vi "Controller Response Matrix Measurement Loop.vi"(7 "Sync Objects":T1, 8 "error in (no error)":errorcluster, 11 "FOFB Configuration":T4={"FOFB Parameters"={"Network"={"FOFB Controller IP"="", "LNLS Control Network IP"="", "LNLS Control Network Power Supplies TCP Port"=0, "LNLS Control Network FOFB Configuration TCP Port"=0, "LNLS Control Network BPMs TCP Port"=0, "Data Server TCP Port"=0, "Monitoring Data TCP Port"=0, "Configuration GUI TCP Port"=0, "Storage Data TCP Port"=0, "TCP Listening Timeout"=0, "Request Setpoints Rate"=0}, "Fast Acquisition"={"Acquisition Period"=0, "Data Buffer Size"=0, "Monitoring Period"=0}, "Response Matrix Measurement"={"Step Amplitude"=0.0, "Time Between Steps"=0, "Step Duration"=0, "Number of Averages"=0}, "Correction Algorithm"={"Correction Period"=0, "Reference Orbit Path"=path "", "Response Matrix Path"=path "", "Correction Matrix Path"=path "", "PID Horizontal Gain"=0.0, "PID Vertical Gain"=0.0, "PID Horizontal Integral Time"=0.0, "PID Vertical Integral Time"=0.0, "PID Horizontal Derivative Time"=0.0, "PID Vertical Derivative Time"=0.0, "Beam Current FOFB Threshold"=0.0, "Decouple H-V"=FALSE, "Use Additional BPM LPF"=FALSE, "BPM LPF Cutoff"=0.0}, "Acquisition Network"=[], "Actuation Network"=[]}, "Number of Acquisition Chassis"=0, "Number of Actuation Chassis"=0, "Number of BPM Readings"=0, "BPM Reading Names"=[], "Selected BPM Readings"=[0, 1, 2, 3, 4, 5, 6, 7, 8, 9, 10, 11, 12, 13, 14, 15, 16, 17, 18, 19, 20, 21, 22, 23, 24, 25, 26, 27, 28, 29, 30, 31, 32, 33, 34, 35, 36, 37, 38, 39, 40, 41, 42, 43, 44, 45, 46, 47, 48, 49], "Number of Correctors"=0, "Corrector Names"=[], "Selected Correctors"=[0, 1, 2, 3, 4, 5, 6, 7, 8, 9, 10, 11, 12, 13, 14, 15, 16, 17, 18, 19, 20, 21, 22, 23, 24, 25, 26, 27, 28, 29, 30, 31, 32, 33, 34, 35, 36, 37, 38, 39, 40, 41, 42, 43, 44, 45, 46, 47, 48, 49], "Reference Orbit"=[], "Response Matrix"=[], "Correction Matrix"=[], "Acquisition Chassis Names"=[], "Actuation Chassis Names"=[], "Acquisition Variables"=[], "Actuation Variables"=[], "PS Matrix Mapping"=[], "Inverse PS Matrix Mapping"=[], "BPM Matrix Mapping"=[], "Inverse BPM Matrix Mapping"=[], "Response Matrix Beam Energy (MeV)"=0.0, "PID Parameters"=[], "BPM Planes"=[], "Corrector Planes"=[], "RMM Step Factor"=[]}) -> (0 "error out":errorcluster)   [LabVIEW 2011, in "Controller VIs.lvlib"]
uses:
  Controller VIs.lvlib
  Types Definitions/Type FOFB Configuration.ctl
  Types Definitions/Type FOFB Parameters.ctl
  Types Definitions/Type Network Configuration.ctl
  Types Definitions/Type FA Configuration.ctl
  Types Definitions/Type Response Matrix Measurement Configuration.ctl
  Types Definitions/Type Correction Algorithm Configuration.ctl
  Types Definitions/Type Acquisition Network Configuration.ctl
  Types Definitions/Type Actuation Network Configuration.ctl
  Types Definitions/Type PID Parameters.ctl
  Types Definitions/Type Synchronization Objects.ctl
  Types Definitions/Type Blocking Synchronization Objects.ctl
  Types Definitions/Type Monitoring Data.ctl
  Types Definitions/Type Operation Mode State.ctl
  Types Definitions/Type Diagnostics Data.ctl
  Types Definitions/Type CPU Loads Array.ctl
  Types Definitions/Type CPU Loads.ctl
  Types Definitions/Type Non-blocking Synchronization Objects.ctl
  Types Definitions/Type FOFB Variables.ctl
  Types Definitions/Type Actuation State.ctl
  <vilib>/Platform/TimedLoop/XDataNode/timing_clust.ctl
  <vilib>/Platform/TimedLoop/XDataNode/nitl_modes.ctl
  <vilib>/Platform/TimedLoop/XDataNode/wakeup.ctl
  Controller Global Variables/Monitoring Data.vi
  <vilib>/Platform/TimedLoop/XDataNode/XDataNode.xnode
  File VIs.lvlib
  Controller Global Variables.lvlib
  Controller Global Variables/LNLS Control FOFB Configuration Out.vi
  <vilib>/Platform/TimedLoop/XDataNode/XDNodeRunTimeDep.lvlib
  Type Definitions.lvlib
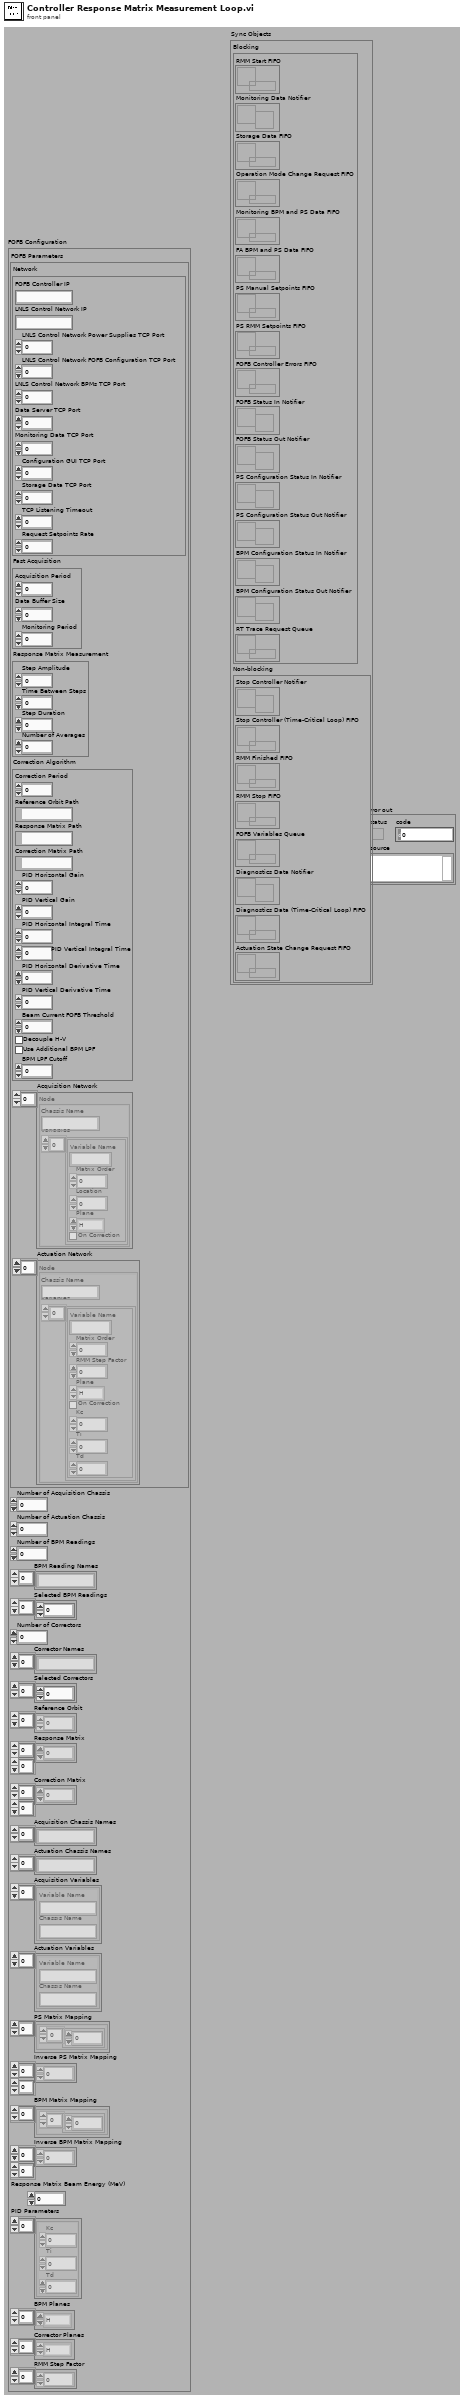
[diagram p1: front panel]
types:
  T1 = typedef "Type Definitions.lvlib/Type Synchronization Objects.ctl" = cluster{"Blocking":T2, "Non-blocking":T3}
  T2 = typedef "Type Definitions.lvlib/Type Blocking Synchronization Objects.ctl" = cluster{"RMM Start FIFO":refnum<k33>, "Monitoring Data Notifier":refnum<notifier>, "Storage Data FIFO":refnum<queue>, "Operation Mode Change Request FIFO":refnum<k33>, "Monitoring BPM and PS Data FIFO":refnum<k33>, "FA BPM and PS Data FIFO":refnum<k33>, "PS Manual Setpoints FIFO":refnum<k33>, "PS RMM Setpoints FIFO":refnum<k33>, "FOFB Controller Errors FIFO ":refnum<k33>, "FOFB Status In Notifier":refnum<notifier>, "FOFB Status Out Notifier":refnum<notifier>, "PS Configuration Status In Notifier":refnum<notifier>, "PS Configuration Status Out Notifier":refnum<notifier>, "BPM Configuration Status In Notifier":refnum<notifier>, "BPM Configuration Status Out Notifier":refnum<notifier>, "RT Trace Request Queue":refnum<queue>}
  T3 = typedef "Type Definitions.lvlib/Type Non-blocking Synchronization Objects.ctl" = cluster{"Stop Controller Notifier":refnum<notifier>, "Stop Controller (Time-Critical Loop) FIFO":refnum<k33>, "RMM Finished FIFO":refnum<k33>, "RMM Stop FIFO":refnum<k33>, "FOFB Variables Queue":refnum<queue>, "Diagnostics Data Notifier":refnum<notifier>, "Diagnostics Data (Time-Critical Loop) FIFO":refnum<k33>, "Actuation State Change Request FIFO":refnum<k33>}
  T4 = typedef "Type Definitions.lvlib/Type FOFB Configuration.ctl" = cluster{"FOFB Parameters":T5, "Number of Acquisition Chassis":i32, "Number of Actuation Chassis":i32, "Number of BPM Readings":i32, "BPM Reading Names":string[], "Selected BPM Readings":u32[], "Number of Correctors":i32, "Corrector Names":string[], "Selected Correctors":u32[], "Reference Orbit":dbl[], "Response Matrix":dbl[][], "Correction Matrix":dbl[][], "Acquisition Chassis Names":string[], "Actuation Chassis Names":string[], "Acquisition Variables":cluster{"Variable Name":string, "Chassis Name":string}[], "Actuation Variables":cluster{"Variable Name":string, "Chassis Name":string}[], "PS Matrix Mapping":cluster{u32[]}[], "Inverse PS Matrix Mapping":u32[][], "BPM Matrix Mapping":cluster{u32[]}[], "Inverse BPM Matrix Mapping":u32[][], "Response Matrix Beam Energy (MeV)":dbl, "PID Parameters":T12[], "BPM Planes":enum8{"H", "V"}[], "Corrector Planes":enum8{"H", "V"}[], "RMM Step Factor":dbl[]}
  T5 = typedef "Type Definitions.lvlib/Type FOFB Parameters.ctl" = cluster{"Network":T6, "Fast Acquisition":T7, "Response Matrix Measurement":T8, "Correction Algorithm":T9, "Acquisition Network":T10, "Actuation Network":T11}
  T6 = typedef "Type Definitions.lvlib/Type Network Configuration.ctl" = cluster{"FOFB Controller IP":string, "LNLS Control Network IP":string, "LNLS Control Network Power Supplies TCP Port":u16, "LNLS Control Network FOFB Configuration TCP Port":u16, "LNLS Control Network BPMs TCP Port":u16, "Data Server TCP Port":u16, "Monitoring Data TCP Port":u16, "Configuration GUI TCP Port":u16, "Storage Data TCP Port":u16, "TCP Listening Timeout":i32, "Request Setpoints Rate":u16}
  T7 = typedef "Type Definitions.lvlib/Type FA Configuration.ctl" = cluster{"Acquisition Period":u32, "Data Buffer Size":u32, "Monitoring Period":u32}
  T8 = typedef "Type Definitions.lvlib/Type Response Matrix Measurement Configuration.ctl" = cluster{"Step Amplitude":dbl, "Time Between Steps":u32, "Step Duration":u32, "Number of Averages":u32}
  T9 = typedef "Type Definitions.lvlib/Type Correction Algorithm Configuration.ctl" = cluster{"Correction Period":u32, "Reference Orbit Path":path, "Response Matrix Path":path, "Correction Matrix Path":path, "PID Horizontal Gain":dbl, "PID Vertical Gain":dbl, "PID Horizontal Integral Time":dbl, "PID Vertical Integral Time":dbl, "PID Horizontal Derivative Time":dbl, "PID Vertical Derivative Time":dbl, "Beam Current FOFB Threshold":dbl, "Decouple H-V":bool, "Use Additional BPM LPF":bool, "BPM LPF Cutoff":dbl}
  T10 = typedef "Type Definitions.lvlib/Type Acquisition Network Configuration.ctl" = cluster{"Chassis Name":string, "Variables":cluster{"Variable Name":string, "Matrix Order":u32, "Location":dbl, "Plane":enum8{"H", "V"}, "On Correction":bool}[]}[]
  T11 = typedef "Type Definitions.lvlib/Type Actuation Network Configuration.ctl" = cluster{"Chassis Name":string, "Variables":cluster{"Variable Name":string, "Matrix Order":u32, "RMM Step Factor":dbl, "Plane":enum8{"H", "V"}, "On Correction":bool, "Kc":dbl, "Ti":dbl, "Td":dbl}[]}[]
  T12 = typedef "Type Definitions.lvlib/Type PID Parameters.ctl" = cluster{"Kc":fxp<+/-,16,8>, "Ti":fxp<+/-,16,8>, "Td":fxp<+/-,16,8>}
  T13 = typedef "XDNodeRunTimeDep.lvlib/timing_clust.ctl" = cluster{"Expected End [f-1]":u64, "Actual End [f-1]":u64, "Finished Late? [f-1]":bool, "Expected End [i-1]":u64, "Actual End [i-1]":u64, "Finished Late? [i-1]":bool, "Expected Start [i]":u64, "Actual Start [i]":u64, "Expected Start [f]":u64, "Actual Start [f]":u64, "Source Name":string, "Structure Name":string, "Period":i64, "Deadline":i64, "Offset":i64, "Start":i64, "Priority":i32, "Timeout":i32, "Mode":T14, "Wakeup Reason":T15, "Error":errorcluster, "Source Type":string, "Secondary Source Type":string, "Global End Time":u64, "Global Start Time":u64, "Frame Duration":u64, "Iteration Duration":u64, "Assigned CPU":i32, "I/O Scan Engine Mode":u32}
  T14 = typedef "XDNodeRunTimeDep.lvlib/nitl_modes.ctl" = enum32{"No Change", "Process missed periods, maintain original phase", "Discard missed periods, maintain original phase", "Process missed periods, ignore original phase", "Discard missed periods, ignore original phase"}
  T15 = typedef "XDNodeRunTimeDep.lvlib/wakeup.ctl" = enum32{"Normal", "Aborted", "Asynchronous wakeup", "Timing source error", "Timed loop error", "Timeout"}
  T16 = typedef "Type Definitions.lvlib/Type Monitoring Data.ctl" = cluster{"Timestamp":timestamp, "BPM Readings":dbl[], "PS Readings":dbl[], "PS FOFB Setpoints":dbl[], "PS Status per Rack":u8[], "PS ON-OFF per Rack":u8[], "Operation Mode":T17, "Diagnostics Data":T18, "Controller Status Table":i32[]}
  T17 = typedef "Type Definitions.lvlib/Type Operation Mode State.ctl" = enum8{"Idle Mode", "Manual Mode", "FOFB Mode", "RMM Mode"}
  T18 = typedef "Type Definitions.lvlib/Type Diagnostics Data.ctl" = cluster{"Time-Critical Loop Missed Iterations":u32, "Time-Critical Loop Execution Time (usec)":u32, "Available Memory (bytes)":u32, "CPU Loads Array":T19}
  T19 = typedef "Type Definitions.lvlib/Type CPU Loads Array.ctl" = T20[]
  T20 = typedef "Type Definitions.lvlib/Type CPU Loads.ctl" = cluster{"Total (%)":dbl, "Time Critical (%)":dbl, "Timed Structures (%)":dbl, "High (%)":dbl, "Above Normal (%)":dbl, "Normal (%)":dbl, "Background (%)":dbl, "Idle (%)":dbl, "ISR (%)":dbl}
  T21 = typedef "Type Definitions.lvlib/Type Control FOFB Configuration Out.ctl" = cluster{"Status":u16, "Operation Mode":T17, "PID Horizontal Gain":sgl, "PID Vertical Gain":sgl, "PID Horizontal Integral Time":sgl, "PID Vertical Integral Time":sgl, "PID Horizontal Derivative Time":sgl, "PID Vertical Derivative Time":sgl, "RMS Horizontal Distortion":dbl, "RMS Vertical Distortion":dbl, "Timestamp":u64}
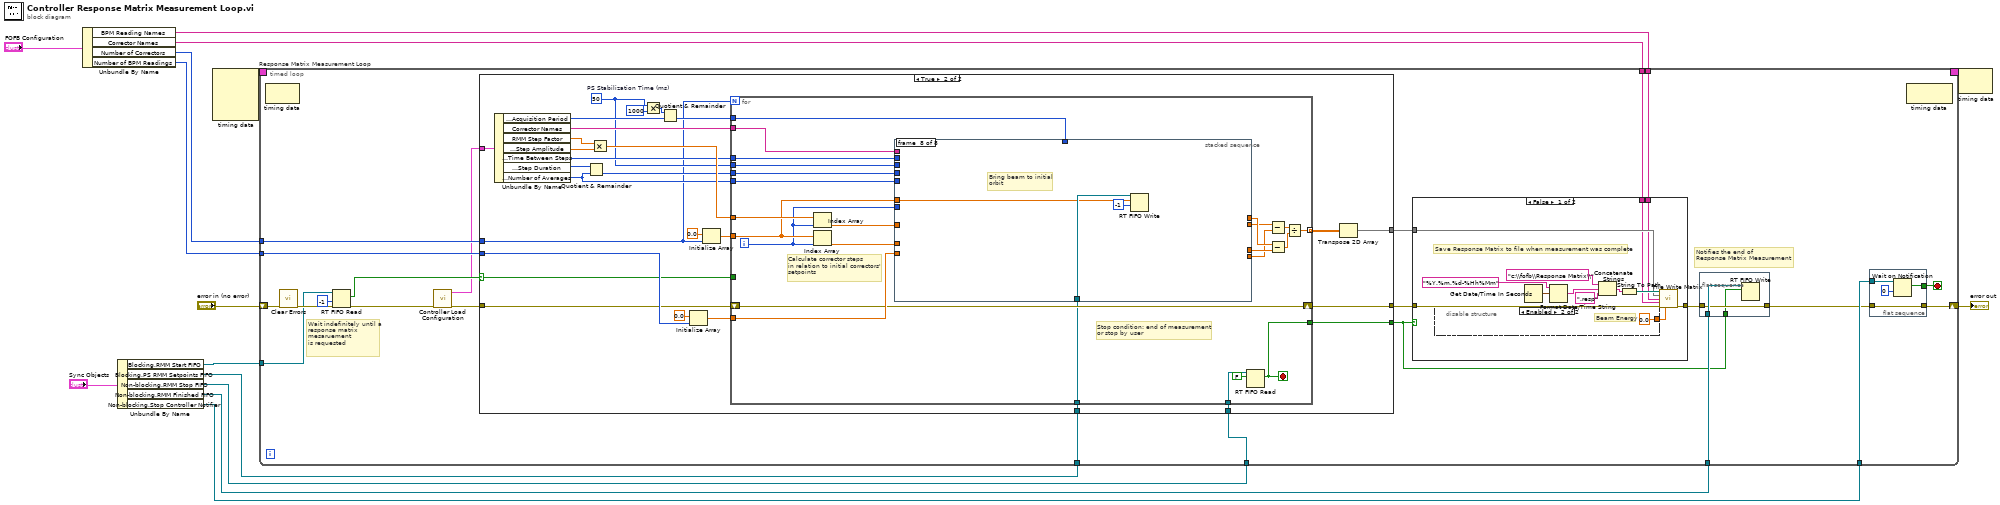
[diagram p0: block diagram]
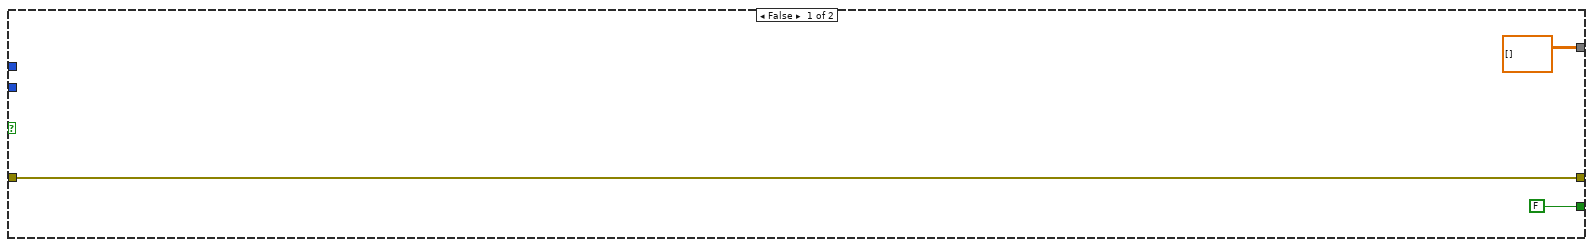
[diagram p2: hidden frame]
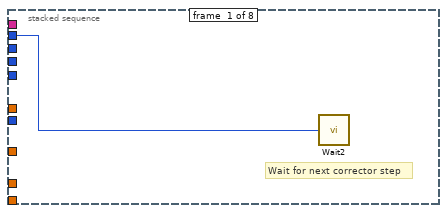
[diagram p3: hidden frame]
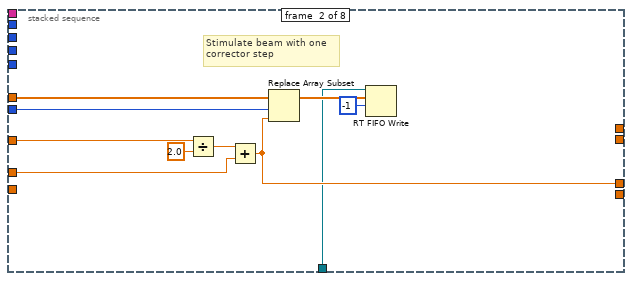
[diagram p4: hidden frame]
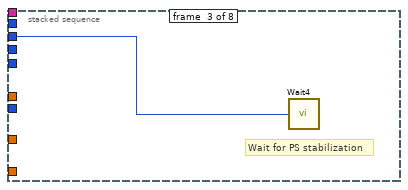
[diagram p5: hidden frame]
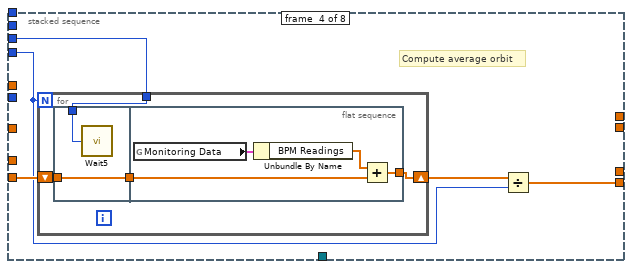
[diagram p6: hidden frame]
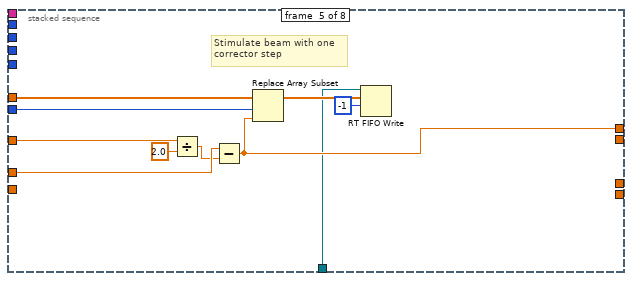
[diagram p7: hidden frame]
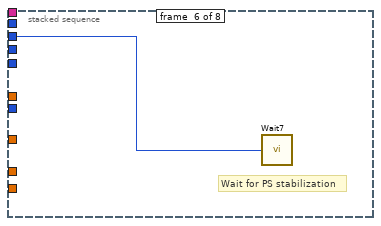
[diagram p8: hidden frame]
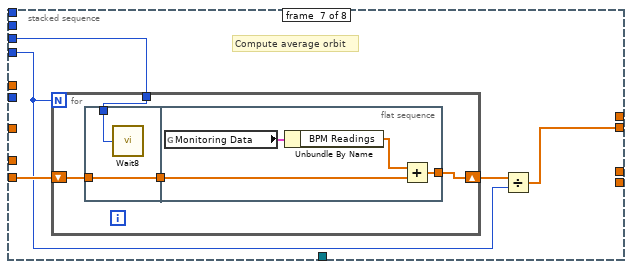
[diagram p9: hidden frame]
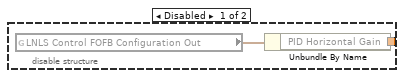
[diagram p10: hidden frame]
diagram:
  n1 = Unbundle By Name("FOFB Configuration") -> ("BPM Reading Names"=w7:string[], "Corrector Names"=w6:string[], "Number of Correctors"=w9:i32, "Number of BPM Readings"=w8:i32)
  n2 = Unbundle By Name("Sync Objects") -> ("Blocking.RMM Start FIFO"=w5:refnum<k33>, "Blocking.PS RMM Setpoints FIFO"=w3:refnum<k33>, "Non-blocking.RMM Stop FIFO"=w10:refnum<k33>, "Non-blocking.RMM Finished FIFO"=w12:refnum<k33>, "Non-blocking.Stop Controller Notifier"=w11:refnum<notifier>)
  n3 = node-c288() -> (w2:T13)  [unwired: 4 in]
  n4 = timed-loop "Response Matrix Measurement Loop" {
    shift-right: [w26] -> w15
    shift-left: "error in (no error)" -> [w21]
    tunnel: w9 -> [w38]
    tunnel: w8 -> [w23]
    tunnel: w7 -> [w37]
    tunnel: w6 -> [w36]
    tunnel: w12 -> [w31]
    tunnel: w11 -> [w35]
    tunnel: w10 -> [w32]
    tunnel: w5 -> [w18]
    tunnel: w3 -> [w24]
    timing: w2 -> [_]
    timing-out: [_] -> w1
    stop <- w27 stop-if-true
    # "Notifies the end of\nResponse Matrix Measurement"
    # "Wait indefinitely until a response matrix mesaruement\nis requested"
    n5 = node-c288() -> ()  [unwired: 1 in, 1 out]
    n6 = call <vilib>:"Clear Errors.vi"("error in (no error)"=w21) -> ("error out"=w19:errorcluster)  [unwired: 6 in]
    n7 = RT FIFO Read(0:w18, 2:-1 ("timeout in ms (-1)"), 3:w19) -> (9:w28:bool, 11:w16:errorcluster)  [unwired: 1 in, 3 out]
    n8 = call "Controller Load Configuration.vi"("error in (no error)"=w16) -> ("error out"=w17:errorcluster, "FOFB Configuration"=w22:T4)  [unwired: 9 in]
    n9 = case shown="True" w28 {
      selector: w28 -> [_ w52]
      tunnel: w17 -> [w50 w66]
      tunnel: [w50 w72] -> w34
      tunnel: [FALSE ("Calculation Stopped?") w71] -> w29
      tunnel: [dbl[][] [] ("Response Matrix") w69] -> w33
      tunnel: w38 -> [_ w51]
      tunnel: w23 -> [_ w68]
      tunnel: w32 -> [_ w63]
      tunnel: w22 -> [_ w62]
      tunnel: w24 -> [_ w59]
      frame False {
      }
      frame True {
        w53 = u32 50  # PS Stabilization Time (ms)
        n10 = Unbundle By Name(w62) -> ("FOFB Parameters.Fast Acquisition.Acquisition Period"=w58:u32, "Corrector Names"=w60:string[], "RMM Step Factor"=w61:dbl[], "FOFB Parameters.Response Matrix Measurement.Step Amplitude"=w77:dbl, "FOFB Parameters.Response Matrix Measurement.Time Between Steps"=w56:u32, "FOFB Parameters.Response Matrix Measurement.Step Duration"=w65:u32, "FOFB Parameters.Response Matrix Measurement.Number of Averages"=w64:u32)
        n11 = Quotient & Remainder(x=w65, y=w64) -> (floor(x/y)=w73:u32)  [unwired: 1 out]
        n12 = Multiply(x=w61, y=w77) -> (x*y=w76:dbl[])
        n13 = Multiply(x=w53, y=u32 1000) -> (x*y=w57:u32)
        n14 = Quotient & Remainder(x=w57, y=w58) -> (floor(x/y)=w54:u32)  [unwired: 1 out]
        n15 = Initialize Array(0.0 ("element"), w68) -> (w74:dbl[])
        n16 = Initialize Array(0.0 ("element"), w51) -> (w67:dbl[])
        n17 = for {
          N: w51 -> [_]
          tunnel: w67 -> [w101]
          tunnel: w76 -> [w102]
          shift-right: [w87] -> w72
          shift-left: w66 -> [w87]
          tunnel: w64 -> [w100]
          tunnel: w74 -> [w99]
          tunnel: w73 -> [w98]
          tunnel: [w86] -> w70 mode=indexing
          tunnel: w56 -> [w89]
          tunnel: [w79] -> w71
          tunnel: w53 -> [w88]
          tunnel: w63 -> [w85]
          tunnel: w60 -> [w84]
          tunnel: w59 -> [w82]
          tunnel: w54 -> [w81]
          tunnel: w52 -> [_]
          i -> [w80]
          stop <- w79 stop-if-true
          # "Stop condition: end of measurement\nor stop by user"
          # "Calculate corrector steps\nin relation to initial correctors'\nsetpoints"
          n18 = Index Array(array=w102, index=w80) -> (element=w91:dbl)
          n19 = Index Array(array=w101, index=w80) -> (element=w90:dbl)
          n20 = stacked-sequence {
            tunnel: w101 -> [_ w109 _ _ w139 _ _ w156]
            tunnel: [_ _ _ _ w133 _ _ _] -> w94
            tunnel: [_ _ _ _ _ _ w141 _] -> w92
            tunnel: w100 -> [_ _ _ w115 _ _ w142 _]
            tunnel: [_ _ _ w118 _ _ _ _] -> w93
            tunnel: [_ w107 _ _ _ _ _ _] -> w95
            tunnel: w99 -> [_ _ _ w117 _ _ w144 _]
            tunnel: w98 -> [_ _ _ w116 _ _ w143 _]
            tunnel: w91 -> [_ w113 _ _ w135 _ _ _]
            tunnel: w90 -> [_ w110 _ _ w137 _ _ _]
            tunnel: w80 -> [_ w108 _ _ w138 _ _ _]
            tunnel: w89 -> [w103 _ _ _ _ _ _ _]
            tunnel: w88 -> [_ _ w114 _ _ w140 _ _]
            tunnel: w84 -> [_ _ _ _ _ _ _ _]
            tunnel: w82 -> [_ w104 _ _ w130 _ _ w157]
            tunnel: w81 -> [_ _ _ _ _ _ _ _]
            frame #0 {
              # "Wait for next corrector step"
              n21 = call "Wait2"("Count(mSec)"=w103) -> ()  [unwired: 1 out]
            }
            frame #1 {
              # "Stimulate beam with one\ncorrector step"
              n22 = Divide(x=w113, y=2.0) -> (x/y=w111:dbl)
              n23 = Add(x=w111, y=w110) -> (x+y=w107:dbl)
              n24 = Replace Array Subset(array=w109, new element=w107, index=w108) -> (w105:dbl[])
              n25 = RT FIFO Write(0:w104, 1:w105, 2:-1 ("timeout in ms (0)")) -> ()  [unwired: 2 in, 4 out]
            }
            frame #2 {
              # "Wait for PS stabilization"
              n26 = call "Wait4"("Count(mSec)"=w114) -> ()  [unwired: 1 out]
            }
            frame #3 {
              # "Compute average orbit"
              n27 = for {
                N: w115 -> [_]
                shift-right: [w121] -> w119
                shift-left: w117 -> [w123]
                tunnel: w116 -> [w120]
                n28 = flat-sequence {
                  tunnel: w123 -> [w125]
                  tunnel: [w125] -> w122
                  tunnel: w120 -> [w124]
                  tunnel: w122 -> [w128]
                  tunnel: [w129] -> w121
                  frame #0 {
                    n29 = call "Wait5"("Count(mSec)"=w124) -> ()  [unwired: 1 out]
                  }
                  frame #1 {
                    n30 = global read "Monitoring Data.vi" "Monitoring Data"() -> (w127:T16)
                    n31 = Unbundle By Name(w127) -> ("BPM Readings"=w126:dbl[])
                    n32 = Add(x=w126, y=w128) -> (x+y=w129:dbl[])
                  }
                }
              }
              n33 = Divide(x=w119, y=w115) -> (x/y=w118:dbl[])
            }
            frame #4 {
              # "Stimulate beam with one\ncorrector step"
              n34 = Divide(x=w135, y=2.0) -> (x/y=w134:dbl)
              n35 = Subtract(x=w137, y=w134) -> (x-y=w133:dbl)
              n36 = Replace Array Subset(array=w139, new element=w133, index=w138) -> (w132:dbl[])
              n37 = RT FIFO Write(0:w130, 1:w132, 2:-1 ("timeout in ms (0)")) -> ()  [unwired: 2 in, 4 out]
            }
            frame #5 {
              # "Wait for PS stabilization"
              n38 = call "Wait7"("Count(mSec)"=w140) -> ()  [unwired: 1 out]
            }
            frame #6 {
              # "Compute average orbit"
              n39 = for {
                N: w142 -> [_]
                shift-right: [w147] -> w145
                shift-left: w144 -> [w149]
                tunnel: w143 -> [w146]
                n40 = flat-sequence {
                  tunnel: w149 -> [w151]
                  tunnel: [w151] -> w148
                  tunnel: w146 -> [w150]
                  tunnel: w148 -> [w154]
                  tunnel: [w155] -> w147
                  frame #0 {
                    n41 = call "Wait8"("Count(mSec)"=w150) -> ()  [unwired: 1 out]
                  }
                  frame #1 {
                    n42 = global read "Monitoring Data.vi" "Monitoring Data"() -> (w153:T16)
                    n43 = Unbundle By Name(w153) -> ("BPM Readings"=w152:dbl[])
                    n44 = Add(x=w152, y=w154) -> (x+y=w155:dbl[])
                  }
                }
              }
              n45 = Divide(x=w145, y=w142) -> (x/y=w141:dbl[])
            }
            frame #7 {
              # "Bring beam to initial\norbit"
              n46 = RT FIFO Write(0:w157, 1:w156, 2:-1 ("timeout in ms (0)")) -> ()  [unwired: 2 in, 4 out]
            }
          }
          n47 = RT FIFO Read(0:w85, 1:FALSE ("element")) -> (9:w79:bool)  [unwired: 2 in, 4 out]
          n48 = Subtract(x=w92, y=w93) -> (x-y=w96:dbl[])
          n49 = Subtract(x=w94, y=w95) -> (x-y=w97:dbl)
          n50 = Divide(x=w96, y=w97) -> (x/y=w86:dbl[])
        }
        n51 = Transpose 2D Array(2D array=w70) -> (transposed array=w69:dbl[][])
      }
    }
    n52 = case shown="False" w29 {
      tunnel: w34 -> [w171 w175]
      tunnel: w33 -> [w165 _]
      tunnel: w37 -> [w162 _]
      tunnel: w36 -> [w161 _]
      tunnel: [w159 w175] -> w30
      frame False {
        # "Save Response Matrix to file when measurement was complete"
        n53 = disable-structure shown="Enabled" {
          disable-tunnel: [w173 0.0 ("Beam Energy (MeV)")] -> w160
          frame Disabled {
            n54 = global read "LNLS Control FOFB Configuration Out.vi" "LNLS Control FOFB Configuration Out"() -> (w172:T21)
            n55 = Unbundle By Name(w172) -> ("PID Horizontal Gain"=w173:sgl)
          }
          frame Enabled {
            # "Beam Energy"
          }
        }
        n56 = Get Date/Time In Seconds() -> (seconds since 1Jan1904=w169:timestamp)
        n57 = Format Date/Time String(time format string (%c)="%Y.%m.%d-%Hh%Mm", seconds (now)=w169) -> (date/time string=w170:string)  [unwired: 1 in]
        n58 = Concatenate Strings("c:\\fofb\\Response Matrix\\", w170, ".resp" ("string")) -> (w167:string)
        n59 = String To Path(string=w167) -> (path=w166:path)
        n60 = call "File Write Matrix.vi"("file path (dialog if empty)"=w166, "Matrix"=w165, "Row Names"=w162, "Column Names"=w161, "error in (no error)"=w171, "Beam Energy (MeV)"=w160) -> ("error out"=w159:errorcluster)  [unwired: 9 in]
      }
      frame True {
        # "If the Response Matrix Measurement was aborted, all data is ignored."
      }
    }
    n61 = flat-sequence {
      tunnel: w31 -> [w47]
      tunnel: w30 -> [w46]
      tunnel: w29 -> [w45]
      tunnel: [w46] -> w25
      frame #0 {
        n62 = RT FIFO Write(0:w47, 1:w45) -> ()  [unwired: 3 in, 4 out]
      }
    }
    n63 = flat-sequence {
      tunnel: w35 -> [w43]
      tunnel: w25 -> [w41]
      tunnel: [w42] -> w27
      tunnel: [w41] -> w26
      frame #0 {
        n64 = Wait on Notification(notifier=w43, timeout in ms (-1)=0) -> (notification=w42:bool)  [unwired: 2 in, 3 out]
      }
    }
    n65 = node-c288() -> ()  [unwired: 1 in, 1 out]
  }
  "error out" <- w15
  n66 = node-c288(w1) -> ()  [unwired: 1 out]
